vi "LabViewLog reader.vi"() -> ()   [LabVIEW 2015]
uses:
  <userlib>/_OpenG.lib/file/file.llb/File Exists - Scalar__ogtk.vi
  <userlib>/_OpenG.lib/file/file.llb/Valid Path - Traditional__ogtk.vi
  source/repos/logReader/Debug/logReader.dll
panel:
  out "return type":string
  out "date":string
  out "file path (use dialog)":path
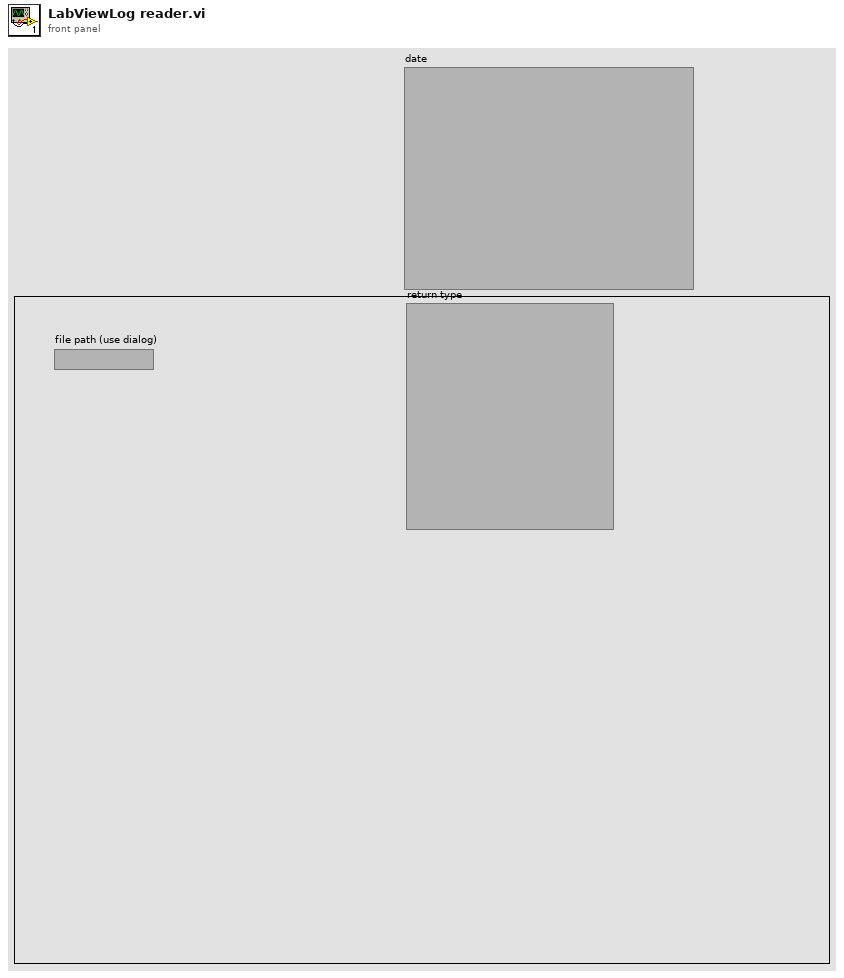
[diagram p1: front panel]
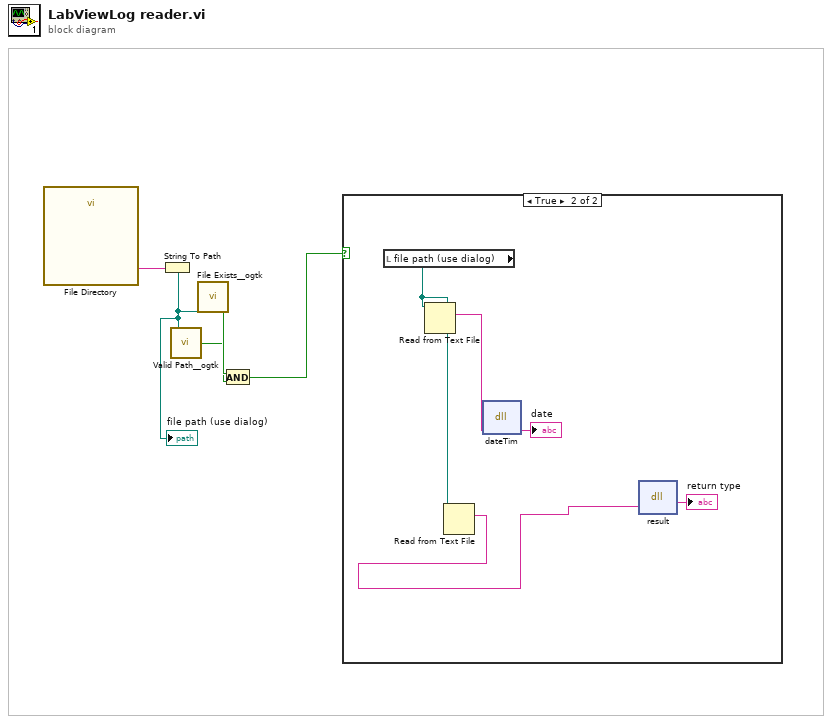
[diagram p0: block diagram]
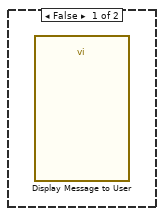
[diagram p2: hidden frame]
diagram:
  n1 = call "File Directory"() -> ("Path:"=w5:string)  [unwired: 17 in, 2 out]
  n2 = String To Path(string=w5) -> (path=w1:path)
  "file path (use dialog)" <- w1
  n3 = call-poly <userlib>:"Valid Path__ogtk.vi"("path"=w1) -> ("valid"=w3:bool)
  n4 = call-poly <userlib>:"File Exists__ogtk.vi"("file path"=w1) -> ("exists"=w4:bool)  [unwired: 6 in, 1 out]
  n5 = And(x=w4, y=w3) -> (x .and. y?=w2:bool)
  n6 = case shown="True" w2 {
    frame False {
      n7 = call "Display Message to User"() -> ()  [unwired: 10 in, 2 out]
    }
    frame True {
      n8 = local read "file path (use dialog)"() -> (w8:path)
      n9 = Read from Text File(file (use dialog)=w8) -> (text=w10:string)  [unwired: 3 in, 3 out]
      n10 = Read from Text File(file (use dialog)=w8) -> (text=w7:string)  [unwired: 3 in, 3 out]
      n11 = dll-call lib="C:/Users/adahal/source/repos/logReader/Debug/logReader.dll" fn="dateTim"("date"=w10) -> ("date"=→"date":string)  [unwired: 4 in, 2 out]
      n12 = dll-call lib="C:/Users/adahal/source/repos/logReader/Debug/logReader.dll" fn="result"("lines"=w7) -> ("return type"=→"return type":string)  [unwired: 4 in, 2 out]
    }
  }
